vi "ALR_init.vi"(0 "Alarms in":T1, 1 "N_param":i32, 5 "fcodealr_full":string[](array[string]), 7 "LevelTable":string[](array[string]), 9 "ALRParameters defs":T4, 11 "error in (no error)":errorcluster, 12 "Names def":string[][](array[string]), 13 "conninfo":T7={"host"="localhost", "port"="5432", "client_encoding"="WIN1251", "dbname"="data", "user"="postgres", "password"=""}, 14 "ALRParamTable":string="f_alr_3") -> (4 "Alarms out":T1, 15 "error":errorcluster)   [LabVIEW 2019, in "Alarms.lvlib"]
uses:
  Alarms.lvlib
  Database/ctl/Coninfo.ctl
  Ctl/ALR_Parameters.ctl
  Ctl/ALR code.ctl
  Ctl/ALR type.ctl
  Ctl/Alarms.ctl
  Ctl/ALR_defs.ctl
  Ctl/ALRs_State.ctl
  Ctl/ALR_ON_OFF.ctl
  Database/PostgreSQL.lvlib
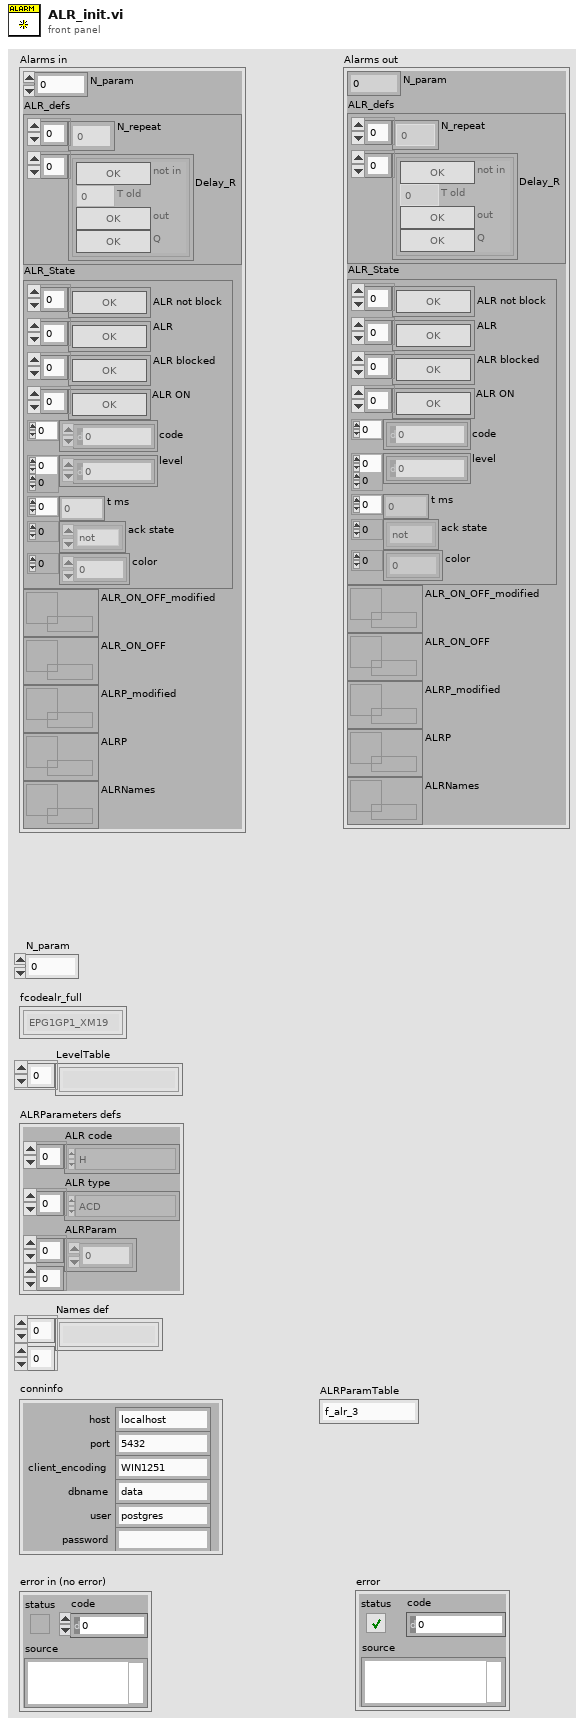
[diagram p1: front panel]
types:
  T1 = typedef "Alarms.lvlib/Alarms.ctl" = cluster{"N_param":i32, "ALR_defs":T2, "ALR_State":T3, "ALR_ON_OFF_modified":refnum<data-value>, "ALR_ON_OFF":refnum<data-value>, "ALRP_modified":refnum<data-value>, "ALRP":refnum<data-value>, "ALRNames":refnum<data-value>}
  T2 = typedef "Alarms.lvlib/ALR_defs.ctl" = cluster{"N_repeat":u32[], "Delay_R":cluster{"not in":bool, "T old":u32, "out":bool, "Q":bool}[]}
  T3 = typedef "Alarms.lvlib/ALRs_State.ctl" = cluster{"ALR not block":bool[], "ALR":bool[], "ALR blocked":bool[], "ALR ON":bool[], "code":i32[], "level":i32[][], "t ms":u32[], "ack state":enum32{"not", "tripped", "reset", "ack"}[], "color":u32[]}
  T4 = typedef "Alarms.lvlib/ALR_Parameters.ctl" = cluster{"ALR code":T5[], "ALR type":T6[], "ALRParam":u32[][]}
  T5 = typedef "Alarms.lvlib/ALR code.ctl" = enum16{"CONN", "H", "HH", "L", "LL", "SERR", "ON", "OFF", "XM19", "XM24", "XM47", "XM51", "XM52", "XM53", "XM54", "XM55", "XM56", "XM61", "XM62", "XM63", "XM64", "XM65", "XM66"}
  T6 = typedef "Alarms.lvlib/ALR type.ctl" = enum16{"ACD", "ACDR", "ALRN", "ALR"}
  T7 = typedef "PostgreSQL.lvlib/Coninfo.ctl" = cluster{"host":string, "port":string, "client_encoding":string, "dbname":string, "user":string, "password":string}
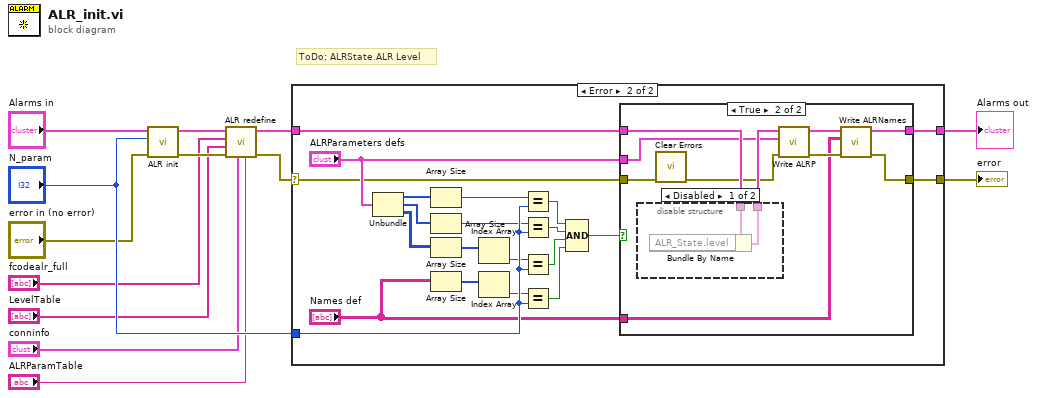
[diagram p0: block diagram]
diagram:
  # "ToDo: ALRState.ALR Level"
  n1 = call "ALR init.vi"("error in (no error)"="error in (no error)", "N_param"="N_param", "Alarms in"="Alarms in") -> ("error out"=w6:errorcluster, "Alarms out"=w8:T1)  [unwired: 7 in]
  n2 = call "ALR redefine.vi"("ALRParamTable"="ALRParamTable", "conninfo"="conninfo", "error in (no error)"=w6, "LevelTable"="LevelTable", "fcodealr_full"="fcodealr_full", "Alarms in"=w8) -> ("error"=w5:errorcluster, "Alarms out"=w7:T1)  [unwired: 4 in]
  n3 = case shown="Error" w5 {
    selector: w5 -> [w15 w18]
    tunnel: "N_param" -> [_ w36]
    tunnel: [w15 w16] -> w13
    tunnel: w7 -> [w14 w22]
    tunnel: [w14 w21] -> w9
    frame No Error {
    }
    frame Error {
      n4 = Unbundle("ALRParameters defs") -> ("ALR code"=w23:T5[], "ALR type"=w24:T6[], "ALRParam"=w25:u32[][])
      n5 = Array Size(array=w23) -> (size(s)=w29:i32)
      n6 = Array Size(array=w24) -> (size(s)=w30:i32)
      n7 = Array Size(array=w25) -> (size(s)=w26:i32[])
      n8 = Array Size(array="Names def") -> (size(s)=w31:i32[])
      n9 = Index Array(array=w26) -> (element=w32:i32)  [unwired: 1 in]
      n10 = Index Array(array=w31) -> (element=w33:i32)  [unwired: 1 in]
      n11 = Equal?(x=w29, y=w36) -> (x = y?=w27:bool)
      n12 = Equal?(x=w30, y=w36) -> (x = y?=w28:bool)
      n13 = Equal?(x=w32, y=w36) -> (x = y?=w34:bool)
      n14 = Equal?(x=w33, y=w36) -> (x = y?=w35:bool)
      n15 = Compound Arithmetic op=AND(w27, w28, w34, w35) -> (w17:bool)
      n16 = case shown="True" w17 {
        tunnel: "Names def" -> [_ w41]
        tunnel: [w37 w43] -> w16
        tunnel: w22 -> [w38 w48]
        tunnel: [w38 w45] -> w21
        tunnel: "ALRParameters defs" -> [_ w42]
        tunnel: w18 -> [w37 w40]
        frame False {
        }
        frame True {
          n17 = disable-structure shown="Disabled" {
            disable-tunnel: w48 -> [w50 w51]
            disable-tunnel: [w49 w51] -> w47
            frame Disabled {
              n18 = Bundle By Name(cluster=w50) -> (w49:T1)  [unwired: 1 in]
            }
            frame Enabled {
            }
          }
          n19 = call <vilib>:"Clear Errors.vi"("error in (no error)"=w40) -> ("error out"=w39:errorcluster)  [unwired: 5 in, 1 out]
          n20 = call "Write ALRP.vi"("error in (no error)"=w39, "ALRP"=w42, "Alarms in"=w47) -> ("error out"=w44:errorcluster, "Alarms out"=w46:T1)  [unwired: 7 in]
          n21 = call "Write ALRNames.vi"("error in (no error)"=w44, "ALRNames"=w41, "Alarms in"=w46) -> ("error out"=w43:errorcluster, "Alarms out"=w45:T1)  [unwired: 7 in]
        }
      }
    }
  }
  "error" <- w13
  "Alarms out" <- w9
